vi "MecaDrivePoseEst_UpdateWithTime.vi"(6 "MecanumWheelPositions":T1 {"RearRight" format="%19.3f"; "RearLeft" format="%19.3f"; "FrontRight" format="%19.3f"; "FrontLeft" format="%19.3f"}, 8 "MecanumWheelSpeeds":T2 {"RearRightSpeed" format="%19.3f"; "RearLeftSpeed" format="%19.3f"; "FrontRightSpeed" format="%19.3f"; "FrontLeftSpeed" format="%19.3f"}, 9 "GyroAngle":T5={"VALUE"=0.0, "COS"=1.0, "SIN"=0.0} {"SIN" format="%13.4f"; "COS" format="%13.4f"; "VALUE" format="%13.4f"}, 10 "CurrentTimeSeconds":dbl, 11 "in MecaDrivePoseEstimate":T6={"M_VisionContR"=[], "m_nominal_dT"=0.0, "m_PrevTime_Sec"=0.0, "m_GyroOffset"={"VALUE"=0.0, "COS"=1.0, "SIN"=0.0}, "m_PrevAngle"={"VALUE"=0.0, "COS"=1.0, "SIN"=0.0}, "m_Observer"={"m_P"=[], "m_xHat"=[], "States"=0, "Outputs"=0, "m_ContR"=[], "m_ContQ"=[], "m_SigmasF"=[], "m_dT_Sec"=0.0, "MERWE_SCALED_SIGMA_PTS"={"m_Wm"=[], "States"=0, "Alpha"=0.0, "m_Wc"=[], "Kappa"=0}, "meanFuncX"=refnum, "meanFuncY"=refnum, "residualFuncX"=refnum, "residualFuncY"=refnum, "addFuncX"=refnum, "addFuncXExtra"=variant, "residualFuncYExtra"=variant, "residualFuncXExtra"=variant, "MeanFuncYExtra"=variant, "MeanFuncXExtra"=variant, "Inputs"=0}, "m_kinematics"={"FrontLeft"={"X"=0.0, "Y"=0.0}, "FrontRight"={"X"=0.0, "Y"=0.0}, "RearLeft"={"X"=0.0, "Y"=0.0}, "RearRight"={"X"=0.0, "Y"=0.0}, "InverseKinematics"=[[0.0, 1.0, -1.0, 0.0], [0.0, 1.0, 1.0, 0.0], [0.0, 1.0, 1.0, 0.0], [0.0, 1.0, -1.0, 0.0]], "ForwardKinematics"=[[0.0, 1.0, -1.0, 0.0], [0.0, 1.0, 1.0, 0.0], [0.0, 1.0, 1.0, 0.0], [0.0, 1.0, -1.0, 0.0]], "PrevCoR"={"X"=0.0, "Y"=0.0}}, "Pose_Buffer"={"TimeStamps"=[], "Pose"=[], "Min_TimeStamp"=0.0, "Max_TimeStamp"=0.0, "ItemCount"=0, "MaxBufferTime"=0.0}} {"Pose_Buffer"."Pose"."ROTATION"."SIN" format="%13.4f"; "Pose_Buffer"."Pose"."ROTATION"."COS" format="%13.4f"; "Pose_Buffer"."Pose"."ROTATION"."VALUE" format="%13.4f"; "Pose_Buffer"."Pose"."TRANSLATION"."Y" format="%14.3f"; "Pose_Buffer"."Pose"."TRANSLATION"."X" format="%14.3f"; "m_kinematics"."PrevCoR"."Y" format="%14.3f"; "m_kinematics"."PrevCoR"."X" format="%14.3f"; "m_kinematics"."RearRight"."Y" format="%14.3f"; "m_kinematics"."RearRight"."X" format="%14.3f"; "m_kinematics"."RearLeft"."Y" format="%14.3f"; "m_kinematics"."RearLeft"."X" format="%14.3f"; "m_kinematics"."FrontRight"."Y" format="%14.3f"; "m_kinematics"."FrontRight"."X" format="%14.3f"; "m_kinematics"."FrontLeft"."Y" format="%14.3f"; "m_kinematics"."FrontLeft"."X" format="%14.3f"; "m_PrevAngle"."SIN" format="%13.4f"; "m_PrevAngle"."COS" format="%13.4f"; "m_PrevAngle"."VALUE" format="%13.4f"; "m_GyroOffset"."SIN" format="%13.4f"; "m_GyroOffset"."COS" format="%13.4f"; "m_GyroOffset"."VALUE" format="%13.4f"}) -> (0 "Error":bool, 2 "Estimated Pose":T3 {"ROTATION"."SIN" format="%13.4f"; "ROTATION"."COS" format="%13.4f"; "ROTATION"."VALUE" format="%13.4f"; "TRANSLATION"."Y" format="%14.3f"; "TRANSLATION"."X" format="%14.3f"}, 3 "Out MecaDrivePoseEstimate":T6={"M_VisionContR"=[], "m_nominal_dT"=0.0, "m_PrevTime_Sec"=0.0, "m_GyroOffset"={"VALUE"=0.0, "COS"=1.0, "SIN"=0.0}, "m_PrevAngle"={"VALUE"=0.0, "COS"=1.0, "SIN"=0.0}, "m_Observer"={"m_P"=[], "m_xHat"=[], "States"=0, "Outputs"=0, "m_ContR"=[], "m_ContQ"=[], "m_SigmasF"=[], "m_dT_Sec"=0.0, "MERWE_SCALED_SIGMA_PTS"={"m_Wm"=[], "States"=0, "Alpha"=0.0, "m_Wc"=[], "Kappa"=0}, "meanFuncX"=refnum, "meanFuncY"=refnum, "residualFuncX"=refnum, "residualFuncY"=refnum, "addFuncX"=refnum, "addFuncXExtra"=variant, "residualFuncYExtra"=variant, "residualFuncXExtra"=variant, "MeanFuncYExtra"=variant, "MeanFuncXExtra"=variant, "Inputs"=0}, "m_kinematics"={"FrontLeft"={"X"=0.0, "Y"=0.0}, "FrontRight"={"X"=0.0, "Y"=0.0}, "RearLeft"={"X"=0.0, "Y"=0.0}, "RearRight"={"X"=0.0, "Y"=0.0}, "InverseKinematics"=[[0.0, 1.0, -1.0, 0.0], [0.0, 1.0, 1.0, 0.0], [0.0, 1.0, 1.0, 0.0], [0.0, 1.0, -1.0, 0.0]], "ForwardKinematics"=[[0.0, 1.0, -1.0, 0.0], [0.0, 1.0, 1.0, 0.0], [0.0, 1.0, 1.0, 0.0], [0.0, 1.0, -1.0, 0.0]], "PrevCoR"={"X"=0.0, "Y"=0.0}}, "Pose_Buffer"={"TimeStamps"=[], "Pose"=[], "Min_TimeStamp"=0.0, "Max_TimeStamp"=0.0, "ItemCount"=0, "MaxBufferTime"=0.0}} {"Pose_Buffer"."Pose"."ROTATION"."SIN" format="%13.4f"; "Pose_Buffer"."Pose"."ROTATION"."COS" format="%13.4f"; "Pose_Buffer"."Pose"."ROTATION"."VALUE" format="%13.4f"; "Pose_Buffer"."Pose"."TRANSLATION"."Y" format="%14.3f"; "Pose_Buffer"."Pose"."TRANSLATION"."X" format="%14.3f"; "m_kinematics"."PrevCoR"."Y" format="%14.3f"; "m_kinematics"."PrevCoR"."X" format="%14.3f"; "m_kinematics"."RearRight"."Y" format="%14.3f"; "m_kinematics"."RearRight"."X" format="%14.3f"; "m_kinematics"."RearLeft"."Y" format="%14.3f"; "m_kinematics"."RearLeft"."X" format="%14.3f"; "m_kinematics"."FrontRight"."Y" format="%14.3f"; "m_kinematics"."FrontRight"."X" format="%14.3f"; "m_kinematics"."FrontLeft"."Y" format="%14.3f"; "m_kinematics"."FrontLeft"."X" format="%14.3f"; "m_PrevAngle"."SIN" format="%13.4f"; "m_PrevAngle"."COS" format="%13.4f"; "m_PrevAngle"."VALUE" format="%13.4f"; "m_GyroOffset"."SIN" format="%13.4f"; "m_GyroOffset"."COS" format="%13.4f"; "m_GyroOffset"."VALUE" format="%13.4f"})   [LabVIEW 2019, in "Trajectory_Library.lvlib"]
doc: "Updates the the Unscented Kalman Filter using only wheel encoder information. This should be called every loop, and the correct loop period must be passed into the constructor of this class.\n \nInputs:\n - SwervePoseEst -- Data cluster containing SwervePoseEst data\n - currentTimeSeconds Time at which this method was called, in seconds.\n - gyroAngle The current gyroscope angle.\n - moduleStates The current velocities and rotations of the swerve modules.\n\nOutputs:\n - outSwevePoseEst -- Updated data cluster \n - EstimatedPose -- The estimated pose of the robot in meters.\n - Error -- If TRUE, an error occured."
uses:
  Trajectory_Library.lvlib
  TypeDef/MECA_DRIVE_POSE_EST.ctl
  <vilib>/Analysis/Matrix/Datatypes/RealMatrix.ctl
  TypeDef/ROTATION2D.ctl
  TypeDef/UNSCENTED_KALMAN_FILTER.ctl
  TypeDef/MERWE_SCALED_SIGMA_PTS.ctl
  TypeDef/CALLBACK_FUNC_TYPE.ctl
  TypeDef/MECA_DRIVE_KINEMATICS.ctl
  TypeDef/TRANSLATION2D.ctl
  TypeDef/TIME_INTERPOLATABLE_POSE2D.ctl
  TypeDef/POSE2D.ctl
  TypeDef/MECA_WHEEL_SPEEDS.ctl
  TypeDef/MECA_WHEEL_POSITIONS.ctl
  Rotation2d_RotateBy.vi
  MatBuilder_Create.vi
  Rotation2d_UnaryMinus.vi
  TimeInterpPose2d_CleanUp.vi
  Rotation2d_CreateXY.vi
  Rotation2d_CreateAngle.vi
  Util_CalcDist.vi
  <vilib>/gmath/interp.llb/Search Ordered Table.vi
  <vilib>/Analysis/Matrix/NI_Matrix.lvlib
panel:
  # "<3, 3>"
  # "State Estimate <Statess,1>"
  # "<States, States>"
  # "<States, ?>"
  # "<Statess,  States>"
  # "<Outputs, Outputs>"
  # "<?, 1>"
  # "<?, 1>"
  # "<3, 3>"
  # "State Estimate <Statess,1>"
  # "<States, States>"
  # "<States, ?>"
  # "<Statess,  States>"
  # "<Outputs, Outputs>"
  # "<?, 1>"
  # "<?, 1>"
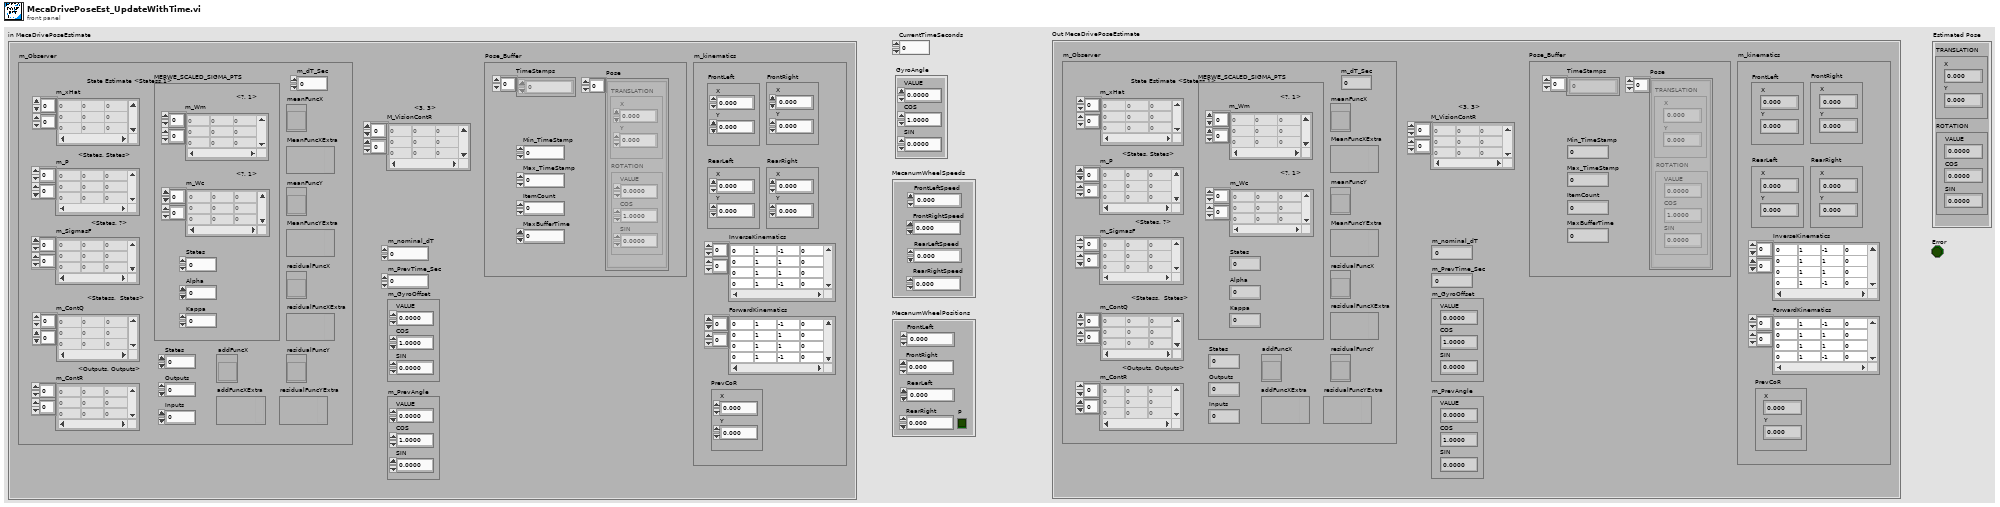
[diagram p1: front panel]
types:
  T1 = typedef "Trajectory_Library.lvlib/MECA_WHEEL_POSITIONS.ctl" = cluster{"FrontLeft":dbl, "FrontRight":dbl, "RearLeft":dbl, "RearRight":dbl, "P":bool}
  T2 = typedef "Trajectory_Library.lvlib/MECA_WHEEL_SPEEDS.ctl" = cluster{"FrontLeftSpeed":dbl, "FrontRightSpeed":dbl, "RearLeftSpeed":dbl, "RearRightSpeed":dbl}
  T3 = typedef "Trajectory_Library.lvlib/POSE2D.ctl" = cluster{"TRANSLATION":T4, "ROTATION":T5}
  T4 = typedef "Trajectory_Library.lvlib/TRANSLATION2D.ctl" = cluster{"X":dbl, "Y":dbl}
  T5 = typedef "Trajectory_Library.lvlib/ROTATION2D.ctl" = cluster{"VALUE":dbl, "COS":dbl, "SIN":dbl}
  T6 = typedef "Trajectory_Library.lvlib/MECA_DRIVE_POSE_EST.ctl" = cluster{"M_VisionContR":T7, "m_nominal_dT":dbl, "m_PrevTime_Sec":dbl, "m_GyroOffset":T5, "m_PrevAngle":T5, "m_Observer":T8, "m_kinematics":T11, "Pose_Buffer":T12}
  T7 = typedef "NI_Matrix.lvlib/RealMatrix.ctl" = dbl[][]
  T8 = typedef "Trajectory_Library.lvlib/UNSCENTED_KALMAN_FILTER.ctl" = cluster{"m_P":T7, "m_xHat":T7, "States":i32, "Outputs":i32, "m_ContR":T7, "m_ContQ":T7, "m_SigmasF":T7, "m_dT_Sec":dbl, "MERWE_SCALED_SIGMA_PTS":T9, "meanFuncX":T10, "meanFuncY":T10, "residualFuncX":T10, "residualFuncY":T10, "addFuncX":T10, "addFuncXExtra":variant, "residualFuncYExtra":variant, "residualFuncXExtra":variant, "MeanFuncYExtra":variant, "MeanFuncXExtra":variant, "Inputs":i32}
  T9 = typedef "Trajectory_Library.lvlib/MERWE_SCALED_SIGMA_PTS.ctl" = cluster{"m_Wm":T7, "States":i32, "Alpha":dbl, "m_Wc":T7, "Kappa":i32}
  T10 = typedef "Trajectory_Library.lvlib/CALLBACK_FUNC_TYPE.ctl" = refnum<vi>
  T11 = typedef "Trajectory_Library.lvlib/MECA_DRIVE_KINEMATICS.ctl" = cluster{"FrontLeft":T4, "FrontRight":T4, "RearLeft":T4, "RearRight":T4, "InverseKinematics":T7, "ForwardKinematics":T7, "PrevCoR":T4}
  T12 = typedef "Trajectory_Library.lvlib/TIME_INTERPOLATABLE_POSE2D.ctl" = cluster{"TimeStamps":dbl[], "Pose":T3[], "Min_TimeStamp":dbl, "Max_TimeStamp":dbl, "ItemCount":i32, "MaxBufferTime":dbl}
  T13 = typedef "Trajectory_Library.lvlib/CHASSIS_SPEEDS.ctl" = cluster{"vX":dbl, "vY":dbl, "vOmega":dbl}
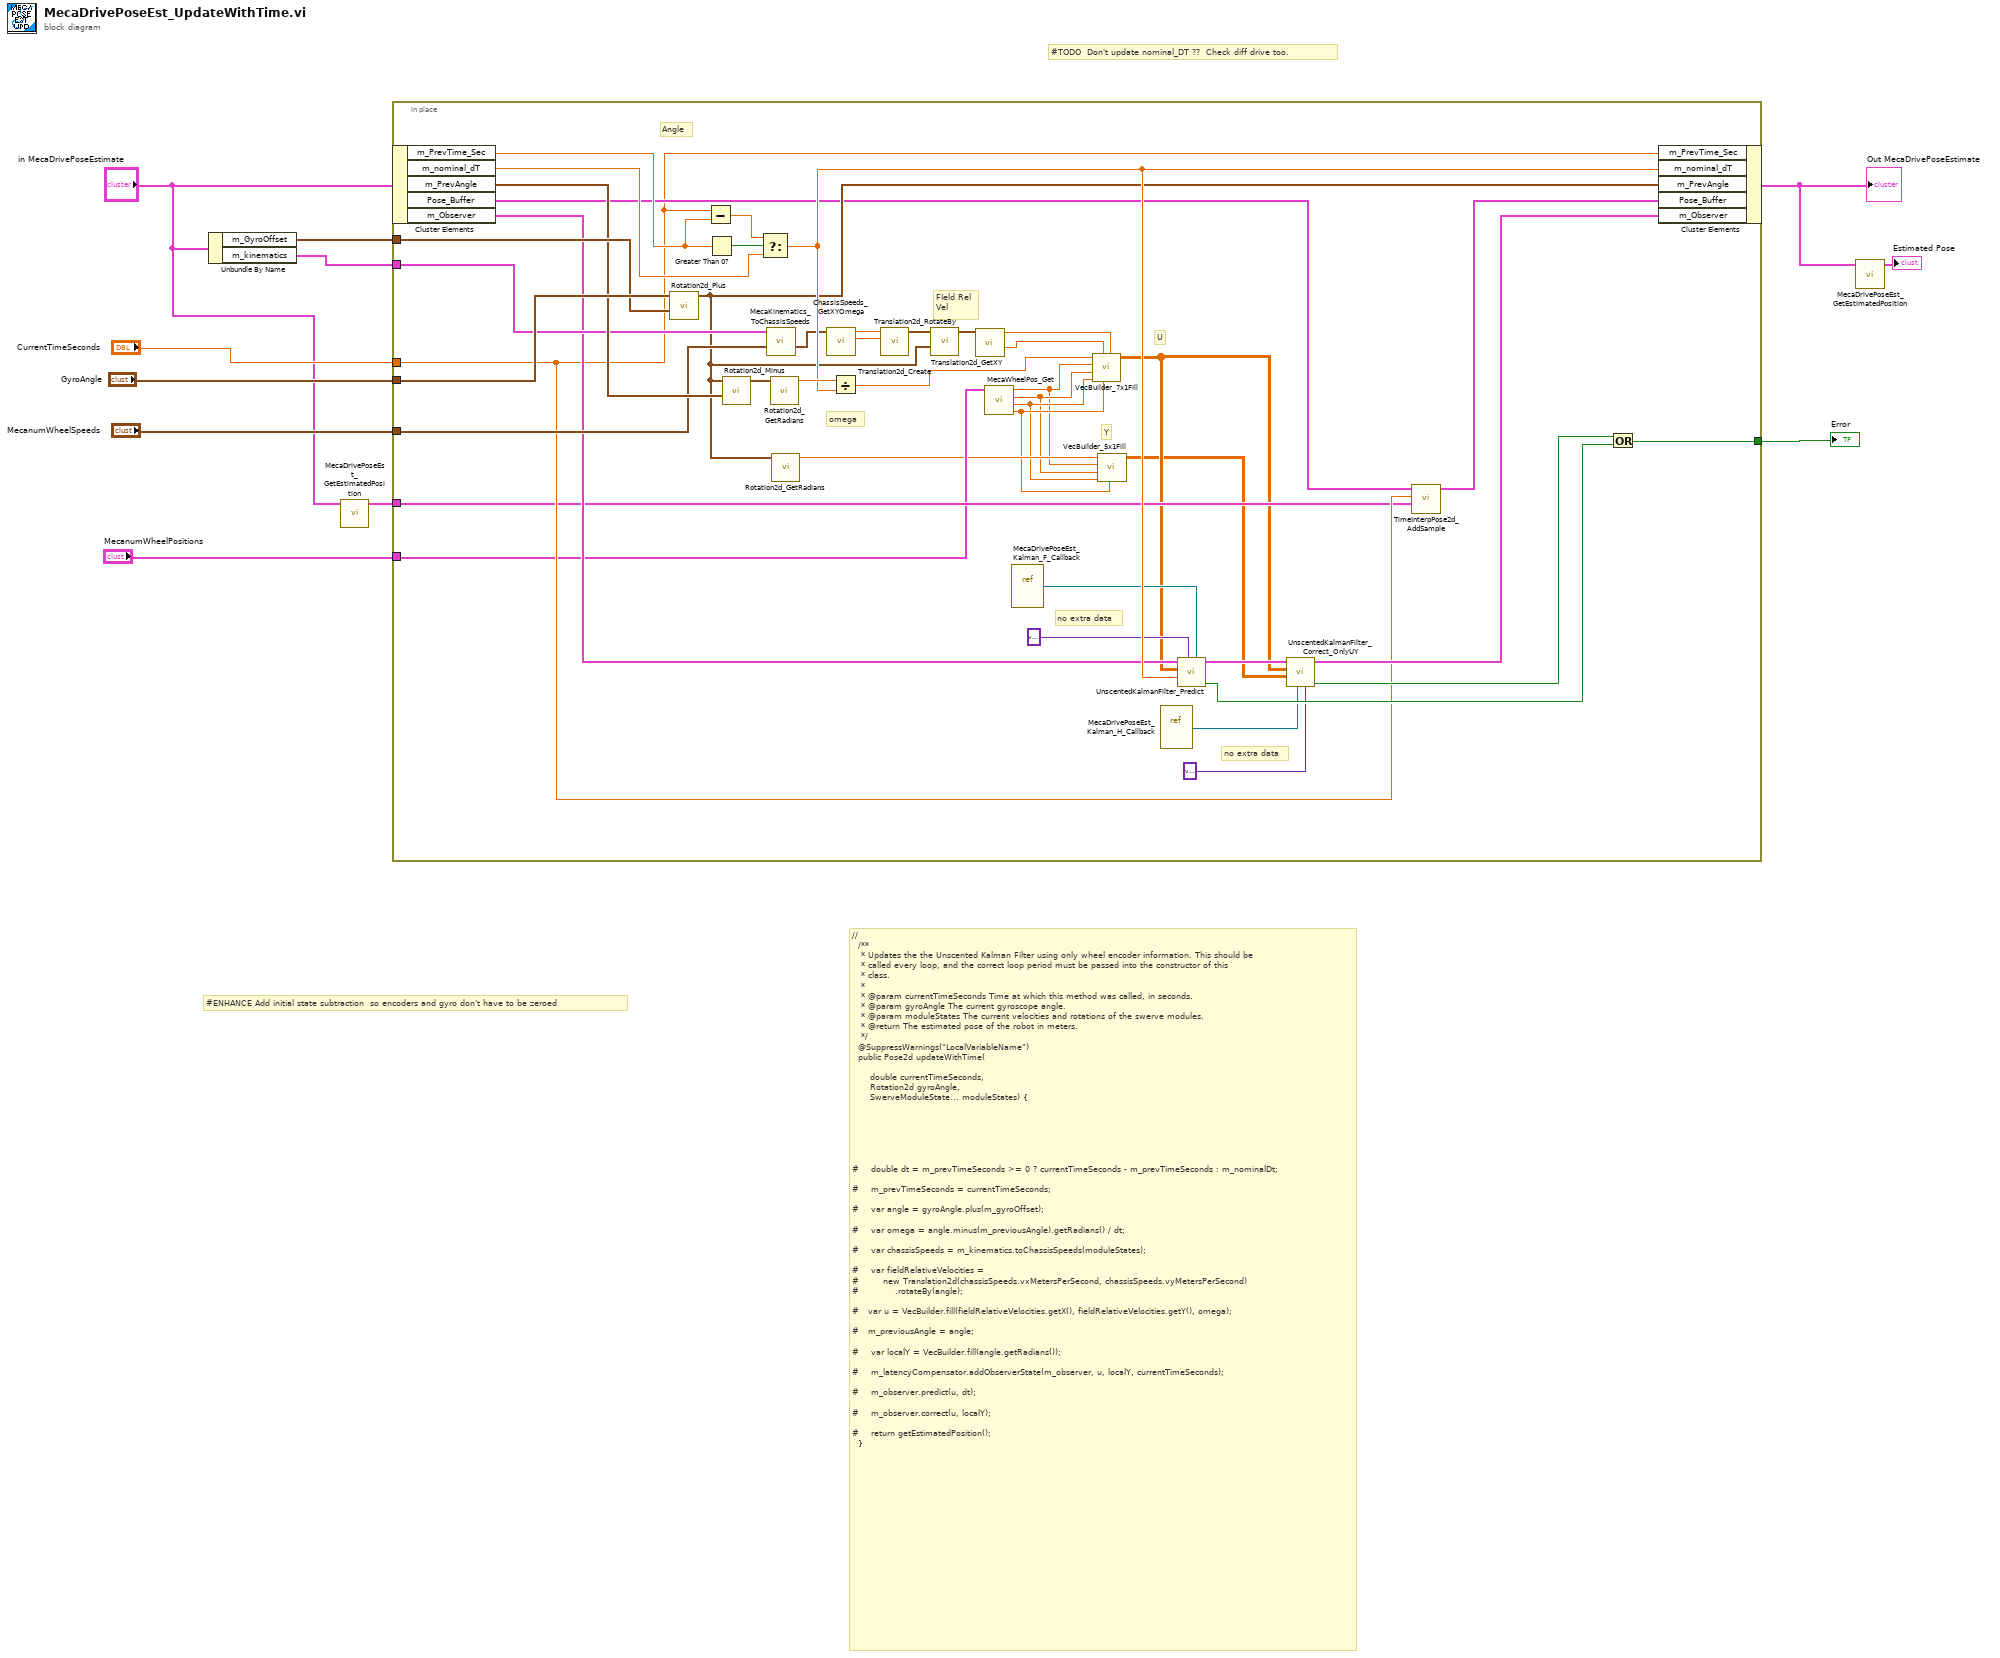
[diagram p0: block diagram]
diagram:
  # "#TODO  Don't update nominal_DT ??  Check diff drive too."
  # "#ENHANCE Add initial state subtraction  so encoders and gyro don't have to be zeroed"
  # "//\n  /**\n   * Updates the the Unscented Kalman Filter using only wheel encoder information. This should be\n   * called every loop, and the correct loop period must be passed into the constructor of this\n   * class.\n   *\n   * @param currentTimeSeconds Time at which this method was called, in seconds.\n   * @param gyroAngle The current gyroscope angle.\n   * @param moduleStates The current velocities and rotations of the swerve modules.\n   * @return The estimated pose of the robot in meters.\n   */\n  @SuppressWarnings(\"LocalVariableName\")\n  public Pose2d updateWithTime(\n\n      double currentTimeSeconds, \n      Rotation2d gyroAngle, \n      SwerveModuleState... moduleStates) {\n\n\n\n\n\n\n#    double dt = m_prevTimeSeconds >= 0 ? currentTimeSeconds - m_prevTimeSeconds : m_nominalDt;\n\n#    m_prevTimeSeconds = currentTimeSeconds;\n\n#    var angle = gyroAngle.plus(m_gyroOffset);\n\n#    var omega = angle.minus(m_previousAngle).getRadians() / dt;\n\n#    var chassisSpeeds = m_kinematics.toChassisSpeeds(moduleStates);\n\n#    var fieldRelativeVelocities =\n#        new Translation2d(chassisSpeeds.vxMetersPerSecond, chassisSpeeds.vyMetersPerSecond)\n#            .rotateBy(angle);\n\n#   var u = VecBuilder.fill(fieldRelativeVelocities.getX(), fieldRelativeVelocities.getY(), omega);\n \n#   m_previousAngle = angle;\n\n#    var localY = VecBuilder.fill(angle.getRadians());\n\n#    m_latencyCompensator.addObserverState(m_observer, u, localY, currentTimeSeconds);\n\n#    m_observer.predict(u, dt);\n\n#    m_observer.correct(u, localY);\n\n#    return getEstimatedPosition();\n  }"
  n1 = Unbundle By Name("in MecaDrivePoseEstimate") -> ("m_GyroOffset"=w9:T5, "m_kinematics"=w5:T11)
  n2 = call "MecaDrivePoseEst_GetEstimatedPosition.vi"("in PoseDrivePoseEstimate"="in MecaDrivePoseEstimate") -> ("Estimated Pose"=w2:T3)  [unwired: 10 in]
  n3 = in-place {
    in-place-border: "CurrentTimeSeconds" -> [w26]
    in-place-border: "GyroAngle" -> [w51]
    in-place-border: w9 -> [w50]
    in-place-border: [w43] -> w6
    in-place-border: w5 -> [w37]
    in-place-border: "MecanumWheelSpeeds" -> [w36]
    in-place-border: w2 -> [w25]
    in-place-border: "MecanumWheelPositions" -> [w21]
    # "FIeld Rel\nVel"
    # "omega"
    # "Angle"
    # "no extra data"
    # "no extra data"
    # "Y"
    # "U"
    n4 = in-place-cluster #1("in MecaDrivePoseEstimate") -> ("m_PrevTime_Sec"=w53:dbl, "m_nominal_dT"=w48:dbl, "m_PrevAngle"=w38:T5, "Pose_Buffer"=w28:T12, "m_Observer"=w29:T8)
    n5 = call "Rotation2d_Plus.vi"("other ROTATION"=w50, "in ROTATION"=w51) -> ("out ROTATION"=w31:T5)  [unwired: 9 in]
    n6 = Subtract(x=w26, y=w53) -> (x-y=w52:dbl)
    n7 = Greater Than 0?(x=w53) -> (x > 0?=w54:bool)
    n8 = call "Rotation2d_Minus.vi"("other ROTATION"=w38, "in ROTATION"=w31) -> ("out ROTATION"=w49:T5)  [unwired: 9 in]
    n9 = Select(t=w52, s=w54, f=w48) -> (s? t:f=w42:dbl)
    n10 = call "MecaKinematics_ToChassisSpeeds.vi"("MECA_WHEEL_SPEEDS"=w36, "in MECA_DRIVE_KINEMATICS"=w37) -> ("ChassisSpeeds"=w35:T13)  [unwired: 9 in]
    n11 = call "Rotation2d_GetRadians.vi"("in ROTATION"=w49) -> ("AngleRadians"=w47:dbl)  [unwired: 10 in]
    n12 = call "Rotation2d_GetRadians.vi"("in ROTATION"=w31) -> ("AngleRadians"=w16:dbl)  [unwired: 10 in]
    n13 = call "ChassisSpeeds_GetXYOmega.vi"("CHASSIS"=w35) -> ("vY"=w33:dbl, "vX"=w34:dbl)  [unwired: 8 in, 1 out]
    n14 = Divide(x=w47, y=w42) -> (x/y=w18:dbl)
    n15 = call "Translation2d_Create.vi"("Y"=w33, "X"=w34) -> ("TRANSLATION"=w32:T4)  [unwired: 9 in]
    n16 = call "Translation2d_RotateBy.vi"("other Rotation"=w31, "In Translation"=w32) -> ("Out Translation"=w30:T4)  [unwired: 9 in]
    n17 = call "Translation2d_GetXY.vi"("In Translation"=w30) -> ("Y"=w19:dbl, "X"=w20:dbl)  [unwired: 9 in]
    n18 = call "MecaWheelPos_Get.vi"("MECA_WHEEL_POSITIONS"=w21) -> ("RearRightPosition"=w15:dbl, "RearLeftPosition"=w14:dbl, "FrontRightPosition"=w13:dbl, "FrontLeftPosition"=w12:dbl)  [unwired: 7 in]
    n19 = vi-ref "MecaDrivePoseEst_Kalman_F_Callback.vi"() -> (w24:refnum<vi>)
    n20 = call "VecBuilder_7x1Fill.vi"("R0"=w20, "R6"=w15, "R1"=w19, "R5"=w14, "R4"=w13, "R3"=w12, "R2"=w18) -> ("output matrix"=w22:T7)  [unwired: 4 in]
    n21 = call "VecBuilder_5x1Fill.vi"("R4"=w15, "R3"=w14, "R2"=w13, "R1"=w12, "R0"=w16) -> ("output matrix"=w17:T7)  [unwired: 6 in]
    n22 = vi-ref "MecaDrivePoseEst_Kalman_H_Callback.vi"() -> (w23:refnum<vi>)
    n23 = call "UnscentedKalmanFilter_Predict.vi"("f_Func"=w24, "F_Func_ExtraData"=variant, "dT_Seconds"=w42, "U"=w22, "in UnscentedKalmanFiilter"=w29) -> ("Error"=w44:bool, "out UnscentedKalmanFiilter"=w46:T8)  [unwired: 5 in]
    n24 = call "UnscentedKalmanFilter_Correct_OnlyUY.vi"("H_ExtraData"=variant ("F_Func_ExtraData"), "H_Func"=w23, "Y"=w17, "U"=w22, "in UnscentedKalmanFiilter"=w46) -> ("Error"=w45:bool, "out UnscentedKalmanFiilter"=w39:T8)  [unwired: 5 in]
    n25 = call "TimeInterpPose2d_AddSample.vi"("Pose"=w25, "TimeStamp"=w26, "in TimeInterpPose"=w28) -> ("out TimeInterpPose"=w27:T12)  [unwired: 7 in, 1 out]
    n26 = Or(x=w45, y=w44) -> (x .or. y?=w43:bool)
    n27 = in-place-cluster #1("m_PrevTime_Sec"=w26, "m_nominal_dT"=w42, "m_PrevAngle"=w31, "Pose_Buffer"=w27, "m_Observer"=w39) -> (w8:T6)
  }
  "Out MecaDrivePoseEstimate" <- w8
  "Error" <- w6
  n28 = call "MecaDrivePoseEst_GetEstimatedPosition.vi"("in PoseDrivePoseEstimate"=w8) -> ("Estimated Pose"=→"Estimated Pose":T3)  [unwired: 10 in]
